vi "Send Launch Nested Actor Msg.vi"(6 "Open Actor Core front panel? (F)":bool, 7 "Message Priority (Normal)":T1=enum."Normal", 8 "error in":errorcluster, 9 "Auto-stop? (T)":bool=TRUE, 10 "Nested Actor":refnum<class "Actor.lvclass">, 11 "Self Enqueuer in":refnum<class "Message Enqueuer.lvclass">) -> (0 "error out":errorcluster, 3 "Self Enqueuer out":refnum<class "Message Enqueuer.lvclass">)   [LabVIEW 2020, in "Actor Framework.lvlib" / "Actor.lvclass"]
doc: "<p>(<strong>Filename</strong>: <span class=\"dnl\">Actor Framework.lvlib:Actor.lvclass:Send Launch Nested Actor Msg.vi</span>)</p>\n\n<p>This VI sends a message containing an actor to another actor. The actor receiving the message will launch the payload actor as a nested actor. Use this VI only to send a message from an actor to itself.</p>"
uses:
  Actor.lvclass
  Launch Nested Actor Msg/Launch Nested Actor Msg.lvclass
  Message Enqueuer/Message Enqueuer.lvclass
  Message Enqueuer/Message Priority.ctl
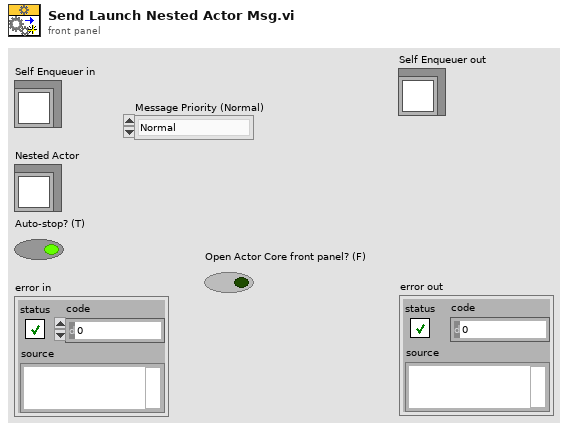
[diagram p1: front panel]
types:
  T1 = typedef "Actor Framework.lvlib/Message Enqueuer.lvclass/Message Priority.ctl" = enum16{"Low", "Normal", "High"}
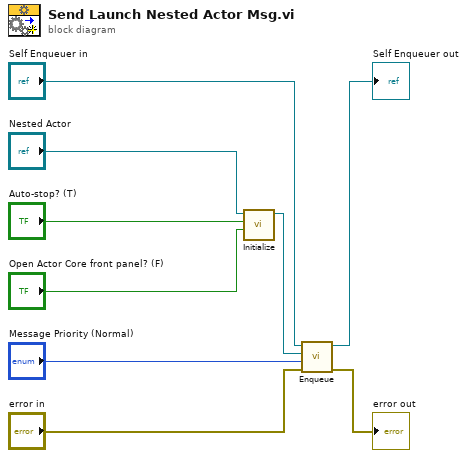
[diagram p0: block diagram]
diagram:
  n1 = call "Initialize.vi"("Open Actor Core front panel? (F)"="Open Actor Core front panel? (F)", "Auto-stop? (T)"="Auto-stop? (T)", "Nested Actor"="Nested Actor") -> ("Launch Nested Actor Msg"=w5:refnum<class "Launch Nested Actor Msg.lvclass">)  [unwired: 8 in]
  n2 = call "Enqueue.vi"("error in (no error)"="error in", "Message Priority (Normal)"="Message Priority (Normal)", "Message"=w5, "Message Enqueuer in"="Self Enqueuer in") -> ("error out"=→"error out":errorcluster, "Message Enqueuer out"=→"Self Enqueuer out":refnum<class "Message Enqueuer.lvclass">)  [unwired: 6 in]
